vi "UMLEditor loadIniFileInfo.vi"(1 "menu":refnum<k9>, 2 "iniFile":path, 5 "error in (no error)":errorcluster) -> (11 "StabilityProblems":bool, 13 "SyncTime":u32, 15 "Ini-FileFound":bool, 16 "ToolHelp":bool, 17 "LastDiagramType":T1, 18 "FileToOpen":path, 19 "error out":errorcluster)   [LabVIEW 2014]
doc: "Gets current diagram values"
uses:
  <resource>/Framework/Providers/Open_GDS/UML/Graph_class/private/diagramType.ctl
  <resource>/Framework/Providers/Open_GDS/UML/UMLEditor/UMLEditor_SyncOptions.ctl
  <resource>/Framework/Providers/Open_GDS/UML/UMLEditor/UMLEditor_IniFileData.ctl
  <resource>/Framework/Providers/Open_GDS/UML/UMLEditor/UMLEditor_StoredPathes.ctl
  <resource>/Framework/Providers/Open_GDS/ClassProviders/Common/File/File_StoredPathesActions.ctl
  <resource>/Framework/Providers/Open_GDS/UML/UMLEditor/UMLEditor_StoredColors.ctl
  <resource>/Framework/Providers/Open_GDS/UML/UmlEditor_class/IniParamsType.ctl
  <resource>/Framework/Providers/Open_GDS/ClassProviders/Common/CommonVIs/CommonVIs_ColorMemoryAction.ctl
  <resource>/Framework/Providers/Open_GDS/UML/UMLEditor/UMLEditor MenuActionType.ctl
  <resource>/Framework/Providers/Open_GDS/UML/Graph_class/Graph.lvclass
  <resource>/Framework/Providers/Open_GDS/UML/UmlEditor_class/UmlEditor.lvclass
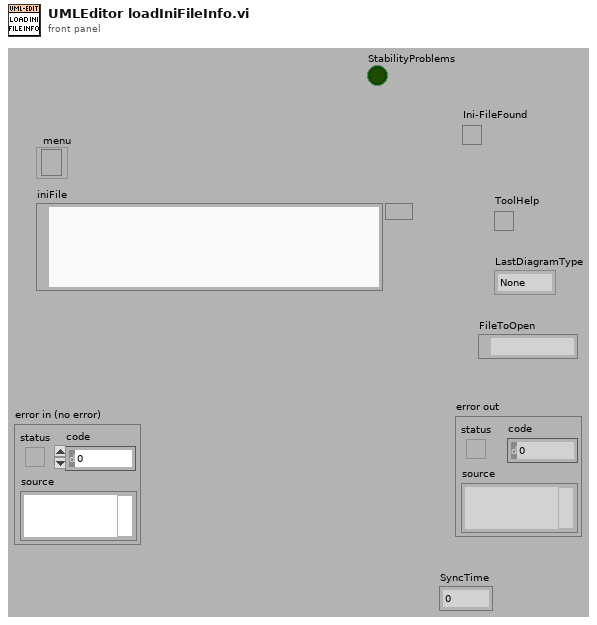
[diagram p1: front panel]
types:
  T1 = typedef "Graph.lvclass/diagramType.ctl" = enum16{"None", "Class", "Sequency", "State", "UseCase"}
  T2 = typedef "UMLEditor_IniFileData.ctl" = cluster{"RecentFiles":string[], "LastDiagramType":T1, "ShowToolHelp":bool, "Paths":cluster{"LastSerachPath":path, "QueuedArrayStateVI":path, "ClassBasePath":path, "VITemplatePath":path, "ApplicationTemplatePath":path, "RevPlugIns":path}, "Colors":cluster{"ClassBackgroudColor":u32, "ClassBackgroudColorWithClassPath":u32, "ClassBackgroudColorForApplicationVIStereotype":u32, "ClassBackgroudColorForTypeStereotype":u32, "StateBackgroudColor":u32}, "ProjectBaseClassOption":bool, "CreateTypesWhenSynchronizing":bool, "AttributeToIgnoreInSync":string[], "ToolTip":cluster{"ToolTipOpen":bool, "LastToolTip":i32}, "ClassesToIgnoreInSync":string[], "UndoSize":i32, "OpenLastSavedFile":bool, "SyncOption":T3, "SyncTime":u32, "Params":cluster{"Name":string, "Value":string}[]}
  T3 = typedef "UMLEditor_SyncOptions.ctl" = cluster{"IgnoreInstrLib":bool, "IgnoreUserLib":bool, "IgnoreViLib":bool}
  T4 = cluster{"RecentFiles":string[], "LastDiagramType":T1, "ShowToolHelp":bool, "Paths":cluster{"LastSerachPath":path, "QueuedArrayStateVI":path, "ClassBasePath":path, "VITemplatePath":path, "ApplicationTemplatePath":path, "RevPlugIns":path}, "Colors":cluster{"ClassBackgroudColor":u32, "ClassBackgroudColorWithClassPath":u32, "ClassBackgroudColorForApplicationVIStereotype":u32, "ClassBackgroudColorForTypeStereotype":u32, "StateBackgroudColor":u32}, "ProjectBaseClassOption":bool, "CreateTypesWhenSynchronizing":bool, "AttributeToIgnoreInSync":string[], "ToolTip":cluster{"ToolTipOpen":bool, "LastToolTip":i32}, "ClassesToIgnoreInSync":string[], "UndoSize":i32, "OpenLastSavedFile":bool, "SyncOption":T3}
  T5 = cluster{"RecentFiles":string[], "LastDiagramType":T1, "ShowToolHelp":bool, "Paths":cluster{"LastSerachPath":path, "QueuedArrayStateVI":path, "ClassBasePath":path, "VITemplatePath":path, "ApplicationTemplatePath":path, "RevPlugIns":path}, "Colors":cluster{"ClassBackgroudColor":u32, "ClassBackgroudColorWithClassPath":u32, "ClassBackgroudColorForApplicationVIStereotype":u32, "ClassBackgroudColorForTypeStereotype":u32, "StateBackgroudColor":u32}, "ProjectBaseClassOption":bool, "CreateTypesWhenSynchronizing":bool, "AttributeToIgnoreInSync":string[], "ToolTip":cluster{"ToolTipOpen":bool, "LastToolTip":i32}, "ClassesToIgnoreInSync":string[], "UndoSize":i32}
  T6 = cluster{"RecentFiles":string[], "LastDiagramType":T1, "ShowToolHelp":bool, "Paths":cluster{"LastSerachPath":path, "QueuedArrayStateVI":path, "ClassBasePath":path, "VITemplatePath":path, "ApplicationTemplatePath":path, "RevPlugIns":path}, "Colors":cluster{"ClassBackgroudColor":u32, "ClassBackgroudColorWithClassPath":u32, "ClassBackgroudColorForApplicationVIStereotype":u32, "ClassBackgroudColorForTypeStereotype":u32, "StateBackgroudColor":u32}, "ProjectBaseClassOption":bool, "CreateTypesWhenSynchronizing":bool, "AttributeToIgnoreInSync":string[], "ToolTip":cluster{"ToolTipOpen":bool, "LastToolTip":i32}, "ClassesToIgnoreInSync":string[], "UndoSize":i32, "OpenLastSavedFile":bool, "SyncOption":T3, "SyncTime":u32}
  T7 = typedef "UmlEditor.lvclass/IniParamsType.ctl" = enum16{"I have problem with UML stability on my computer"}
  T8 = typedef "UMLEditor_StoredColors.ctl" = enum16{"ClassBackgroudColor", "ClassBackgroudColorWithClassPath", "ClassBackgroudColorForApplicationVIStereotype", "ClassBackgroudColorForTypeStereotype", "StateBackgroudColor"}
  T9 = typedef "UMLEditor_StoredPathes.ctl" = enum16{"LastSearchPath", "QueuedArrayStateVI", "ClassBasePath", "ViTemplatePath", "ApplicationTemplatePath", "IniFilePath", "WizDir", "RevPlugInPath"}
  T10 = typedef "UMLEditor MenuActionType.ctl" = enum16{"EnableSave", "EnablePaste", "DisablePaste", "DiableSave", "AddRecentFile", "disablePropDel", "enablePropDel", "enablePropDisDel", "diasbleClassRel", "enableClassRel", "Class", "State", "Other", "EnableXMI", "DisableXMI"}
  T11 = typedef "CommonVIs_ColorMemoryAction.ctl" = enum16{"Get Color", "Set Color", "Delete Color", "Clear All Colors"}
  T12 = typedef "File_StoredPathesActions.ctl" = enum16{"Get Path", "Set Path", "Delete Path", "Clear All Paths"}
  T13 = cluster{"LastSerachPath":path, "QueuedArrayStateVI":path, "ClassBasePath":path, "VITemplatePath":path, "ApplicationTemplatePath":path, "RevPlugIns":path}
  T14 = cluster{"ClassBackgroudColor":u32, "ClassBackgroudColorWithClassPath":u32, "ClassBackgroudColorForApplicationVIStereotype":u32, "ClassBackgroudColorForTypeStereotype":u32, "StateBackgroudColor":u32}
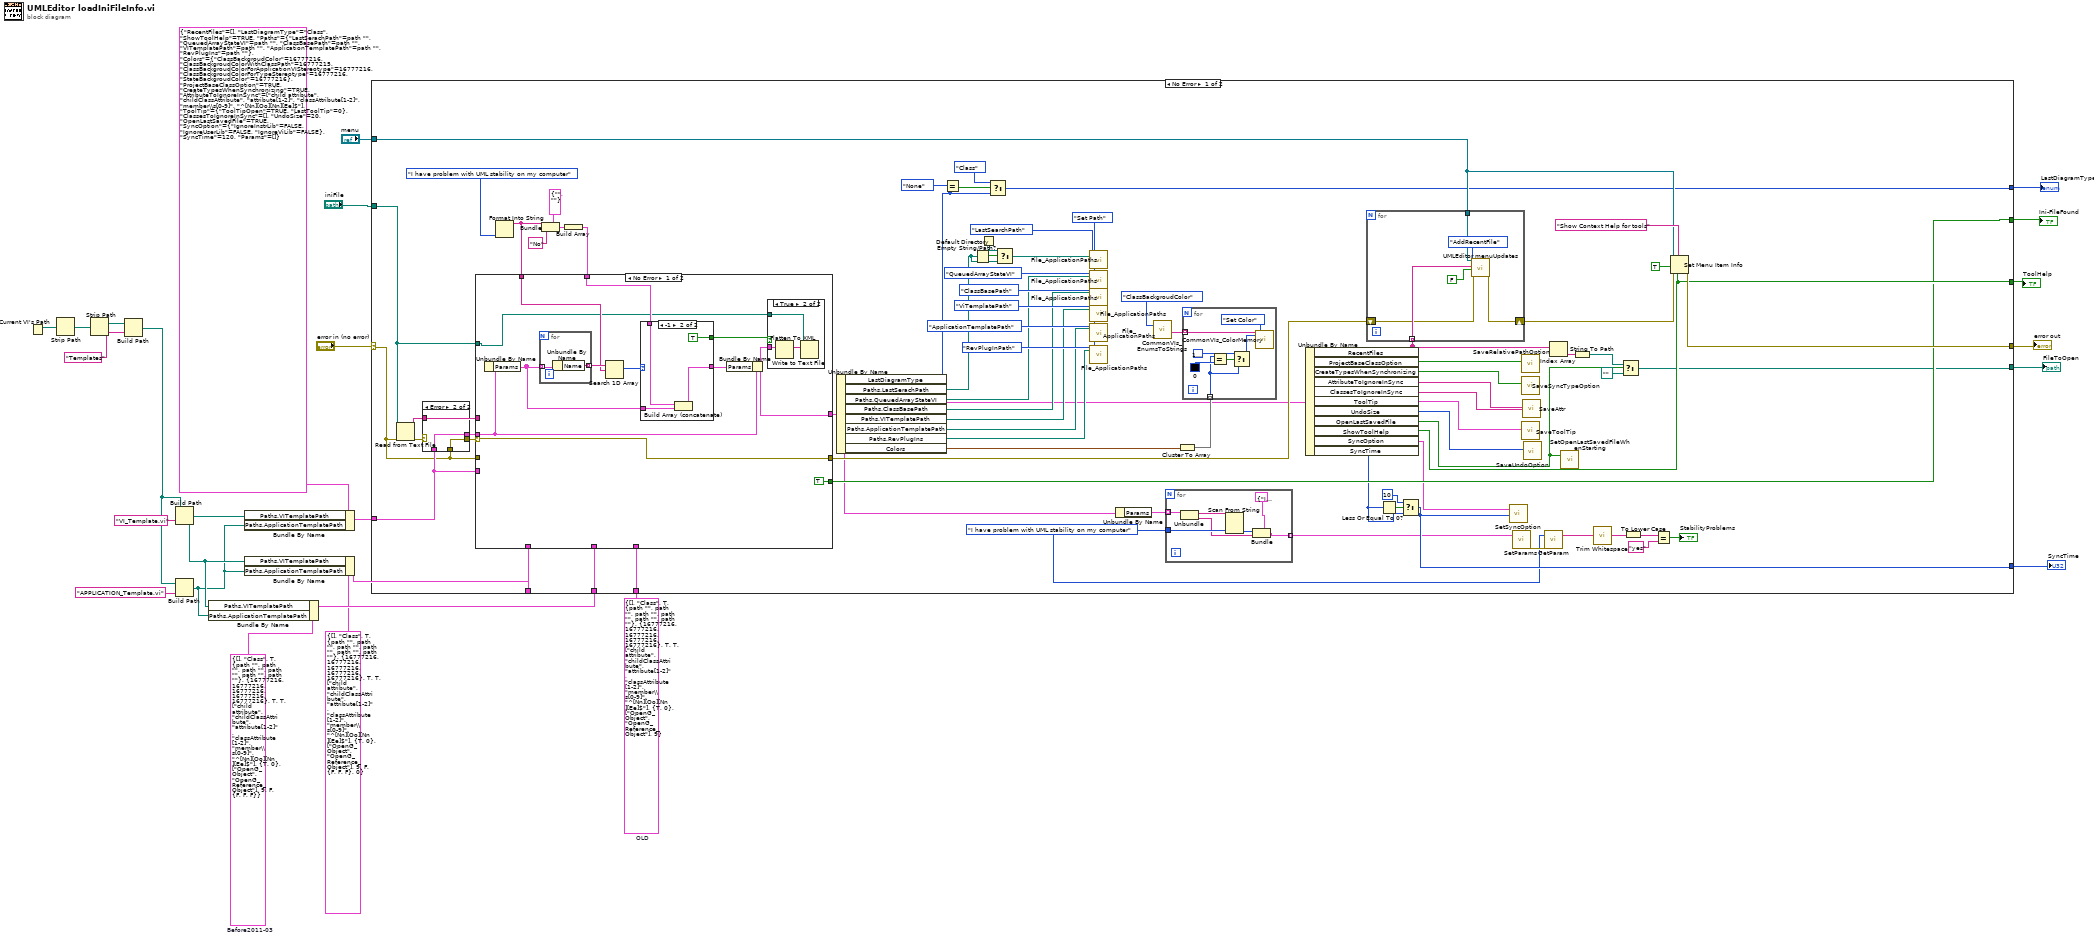
[diagram p0: block diagram]
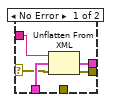
[diagram p2: hidden frame]
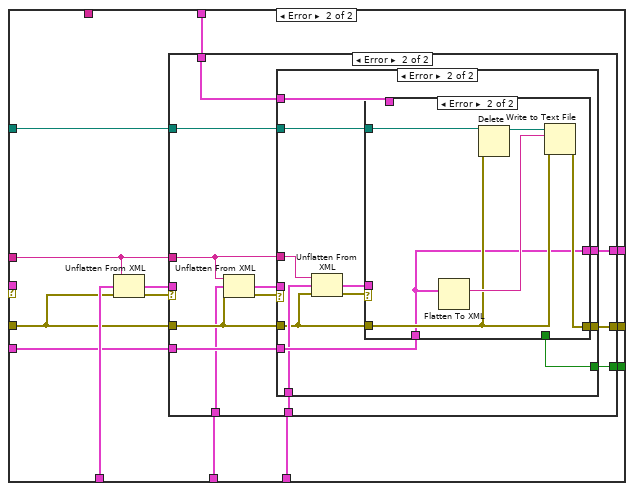
[diagram p5: hidden frame]
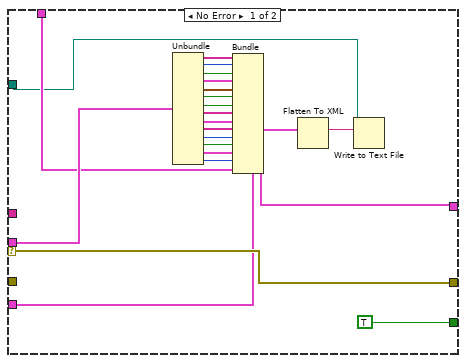
[diagram p6: hidden frame]
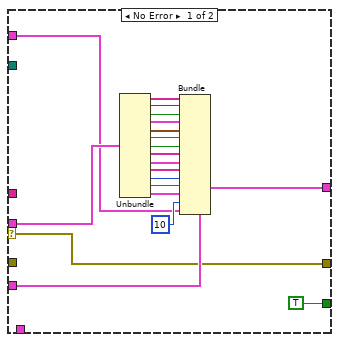
[diagram p7: hidden frame]
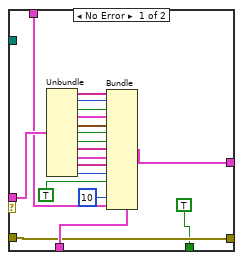
[diagram p8: hidden frame]
diagram:
  w9 = T4 {"RecentFiles"=[], "LastDiagramType"=enum."Class", "ShowToolHelp"=TRUE, "Paths"={"LastSerachPath"=path "", "QueuedArrayStateVI"=path "", "ClassBasePath"=path "", "VITemplatePath"=path "", "ApplicationTemplatePath"=path "", "RevPlugIns"=path ""}, "Colors"={"ClassBackgroudColor"=16777216, "ClassBackgroudColorWithClassPath"=16777216, "ClassBackgroudColorForApplicationVIStereotype"=16777216, "ClassBackgroudColorForTypeStereotype"=16777216, "StateBackgroudColor"=16777216}, "ProjectBaseClassOption"=TRUE, "CreateTypesWhenSynchronizing"=TRUE, "AttributeToIgnoreInSync"=["child attribute", "childClassAttribute", "attribute[1-2]", "classAttribute[1-2]", "member\\s[0-9]", "^[Nn][Oo][Nn][Ee]$"], "ToolTip"={"ToolTipOpen"=TRUE, "LastToolTip"=0}, "ClassesToIgnoreInSync"=["OpenG_Object", "OpenG_Reference_Object"], "UndoSize"=9, "OpenLastSavedFile"=FALSE, "SyncOption"={"IgnoreInstrLib"=FALSE, "IgnoreUserLib"=FALSE, "IgnoreViLib"=FALSE}}  # Before2011-03
  w11 = T5 {"RecentFiles"=[], "LastDiagramType"=enum."Class", "ShowToolHelp"=TRUE, "Paths"={"LastSerachPath"=path "", "QueuedArrayStateVI"=path "", "ClassBasePath"=path "", "VITemplatePath"=path "", "ApplicationTemplatePath"=path "", "RevPlugIns"=path ""}, "Colors"={"ClassBackgroudColor"=16777216, "ClassBackgroudColorWithClassPath"=16777216, "ClassBackgroudColorForApplicationVIStereotype"=16777216, "ClassBackgroudColorForTypeStereotype"=16777216, "StateBackgroudColor"=16777216}, "ProjectBaseClassOption"=TRUE, "CreateTypesWhenSynchronizing"=TRUE, "AttributeToIgnoreInSync"=["child attribute", "childClassAttribute", "attribute[1-2]", "classAttribute[1-2]", "member\\s[0-9]", "^[Nn][Oo][Nn][Ee]$"], "ToolTip"={"ToolTipOpen"=TRUE, "LastToolTip"=0}, "ClassesToIgnoreInSync"=["OpenG_Object", "OpenG_Reference_Object"], "UndoSize"=9}  # OLD
  n1 = Current VI's Path() -> (path=w18:path)
  n2 = Strip Path(path=w18) -> (stripped path=w17:path)  [unwired: 1 out]
  n3 = Strip Path(path=w17) -> (stripped path=w16:path)  [unwired: 1 out]
  n4 = Build Path(base path=w16, name or relative path="Templates") -> (appended path=w14:path)
  n5 = Build Path(base path=w14, name or relative path="VI_Template.vi") -> (appended path=w5:path)
  n6 = Build Path(base path=w14, name or relative path="APPLICATION_Template.vi") -> (appended path=w4:path)
  n7 = Bundle By Name(cluster=w9, "Paths.VITemplatePath"=w5, "Paths.ApplicationTemplatePath"=w4) -> (w8:T4)
  n8 = Bundle By Name(cluster=T2 {"RecentFiles"=[], "LastDiagramType"=enum."Class", "ShowToolHelp"=TRUE, "Paths"={"LastSerachPath"=path "", "QueuedArrayStateVI"=path "", "ClassBasePath"=path "", "VITemplatePath"=path "", "ApplicationTemplatePath"=path "", "RevPlugIns"=path ""}, "Colors"={"ClassBackgroudColor"=16777216, "ClassBackgroudColorWithClassPath"=16777215, "ClassBackgroudColorForApplicationVIStereotype"=16777216, "ClassBackgroudColorForTypeStereotype"=16777216, "StateBackgroudColor"=16777216}, "ProjectBaseClassOption"=TRUE, "CreateTypesWhenSynchronizing"=TRUE, "AttributeToIgnoreInSync"=["child attribute", "childClassAttribute", "attribute[1-2]", "classAttribute[1-2]", "member\\s[0-9]", "^[Nn][Oo][Nn][Ee]$"], "ToolTip"={"ToolTipOpen"=TRUE, "LastToolTip"=0}, "ClassesToIgnoreInSync"=[], "UndoSize"=20, "OpenLastSavedFile"=TRUE, "SyncOption"={"IgnoreInstrLib"=FALSE, "IgnoreUserLib"=FALSE, "IgnoreViLib"=FALSE}, "SyncTime"=120, "Params"=[]} ("INiFileData"), "Paths.VITemplatePath"=w5, "Paths.ApplicationTemplatePath"=w4) -> (w3:T2)
  n9 = Bundle By Name(cluster=T6 {"RecentFiles"=[], "LastDiagramType"=enum."Class", "ShowToolHelp"=TRUE, "Paths"={"LastSerachPath"=path "", "QueuedArrayStateVI"=path "", "ClassBasePath"=path "", "VITemplatePath"=path "", "ApplicationTemplatePath"=path "", "RevPlugIns"=path ""}, "Colors"={"ClassBackgroudColor"=16777216, "ClassBackgroudColorWithClassPath"=16777216, "ClassBackgroudColorForApplicationVIStereotype"=16777216, "ClassBackgroudColorForTypeStereotype"=16777216, "StateBackgroudColor"=16777216}, "ProjectBaseClassOption"=TRUE, "CreateTypesWhenSynchronizing"=TRUE, "AttributeToIgnoreInSync"=["child attribute", "childClassAttribute", "attribute[1-2]", "classAttribute[1-2]", "member\\s[0-9]", "^[Nn][Oo][Nn][Ee]$"], "ToolTip"={"ToolTipOpen"=TRUE, "LastToolTip"=0}, "ClassesToIgnoreInSync"=["OpenG_Object", "OpenG_Reference_Object"], "UndoSize"=9, "OpenLastSavedFile"=FALSE, "SyncOption"={"IgnoreInstrLib"=FALSE, "IgnoreUserLib"=FALSE, "IgnoreViLib"=FALSE}, "SyncTime"=0} ("INiFileData"), "Paths.VITemplatePath"=w5, "Paths.ApplicationTemplatePath"=w4) -> (w19:T6)
  n10 = case shown="No Error" "error in (no error)" {
    selector: "error in (no error)" -> [w26 w254]
    tunnel: [w101 w254] -> w24
    tunnel: [w64 _] -> w23
    tunnel: [w70 _] -> w22
    tunnel: [w80 _] -> w21
    tunnel: "menu" -> [w95 _]
    tunnel: "iniFile" -> [w81 _]
    tunnel: w19 -> [w82 _]
    tunnel: w11 -> [w60 _]
    tunnel: [w54 _] -> w10
    tunnel: w8 -> [w52 _]
    tunnel: [w49 _] -> w7
    tunnel: w3 -> [w44 _]
    frame No Error {
      w34 = IniParamsType."I have problem with UML stability on my computer" ("IniParams")
      w85 = File_StoredPathesActions."Set Path" ("Method (Get Path)")
      n11 = Read from Text File(file (use dialog)=w81, error in=w26) -> (text=w47:string, error out=w27:errorcluster)  [unwired: 4 out]
      n12 = case shown="Error" w27 {
        selector: w27 -> [w102 _]
        tunnel: w47 -> [w106 _]
        tunnel: [w105 w107] -> w46
        tunnel: [w104 w108] -> w45
        tunnel: w44 -> [w103 w108]
        tunnel: w26 -> [_ w107]
        frame No Error {
          n13 = Unflatten From XML(xml string=w106, type=w103, error in (no error)=w102) -> (value=w104:T2, error out=w105:errorcluster)
        }
        frame Error {
        }
      }
      n14 = Format Into String(IniParamsType."I have problem with UML stability on my computer" ("IniParams")) -> (resulting string=w28:string)  [unwired: 3 in, 1 out]
      n15 = Bundle(cluster=cluster{"Name":string, "Value":string} {"Name"="", "Value"=""} ("Param"), "Name"=w28, "Value"="No") -> (w40:cluster{"Name":string, "Value":string})
      n16 = Build Array(w40) -> (w39:cluster{"Name":string, "Value":string}[])
      n17 = case shown="No Error" w46 {
        selector: w46 -> [w127 _]
        tunnel: w26 -> [_ w140]
        tunnel: w82 -> [_ w149]
        tunnel: w81 -> [w117 w148]
        tunnel: [w127 w146] -> w69
        tunnel: [TRUE w145] -> w64
        tunnel: w60 -> [_ w144]
        tunnel: [w116 w143] -> w38
        tunnel: w52 -> [_ w142]
        tunnel: w47 -> [_ w141]
        tunnel: w45 -> [w123 _]
        tunnel: w44 -> [_ w139]
        tunnel: w39 -> [w120 w138]
        tunnel: w28 -> [w124 _]
        frame No Error {
          n18 = Unbundle By Name(w123) -> ("Params"=w121:cluster{"Name":string, "Value":string}[])
          n19 = for {
            tunnel: w121 -> [w137] mode=indexing
            tunnel: [w136] -> w125 mode=indexing
            n20 = Unbundle By Name(w137) -> ("Name"=w136:string)
          }
          n21 = Search 1D Array(1D array=w125, element=w124) -> (index of element=w122:i32)  [unwired: 1 in]
          n22 = case shown="-1" w122 {
            tunnel: w121 -> [w131 w135]
            tunnel: w120 -> [_ w134]
            tunnel: [w131 w133] -> w119
            tunnel: [_ TRUE] -> w118
            frame 0, Default {
            }
            frame -1 {
              n23 = Build Array (concatenate)(w134, w135) -> (w133:cluster{"Name":string, "Value":string}[])
            }
          }
          n24 = Bundle By Name(cluster=w123, "Params"=w119) -> (w116:T2)
          n25 = case shown="True" w118 {
            tunnel: w117 -> [_ w129]
            tunnel: w116 -> [_ w128]
            frame False {
            }
            frame True {
              n26 = Flatten To XML(anything=w128) -> (xml string=w130:string)
              n27 = Write to Text File(file (use dialog)=w129, text=w130) -> ()  [unwired: 1 in, 4 out]
            }
          }
        }
        frame Error {
          n28 = Unflatten From XML(xml string=w141, type=w149, error in (no error)=w140) -> (value=w147:T6, error out=w150:errorcluster)
          n29 = case shown="Error" w150 {
            selector: w150 -> [w172 _]
            tunnel: [w172 w182] -> w146
            tunnel: w140 -> [_ w178]
            tunnel: w139 -> [w155 w183]
            tunnel: w148 -> [w151 w184]
            tunnel: w147 -> [w157 _]
            tunnel: [TRUE w181] -> w145
            tunnel: w141 -> [_ w177]
            tunnel: w144 -> [_ w180]
            tunnel: [w153 w179] -> w143
            tunnel: w142 -> [_ w174]
            tunnel: w138 -> [w154 w173]
            frame No Error {
              n30 = Unbundle(w157) -> ("RecentFiles"=w170:string[], "LastDiagramType"=w169:T1, "ShowToolHelp"=w168:bool, "Paths"=w167:T13, "Colors"=w166:T14, "ProjectBaseClassOption"=w165:bool, "CreateTypesWhenSynchronizing"=w164:bool, "AttributeToIgnoreInSync"=w163:string[], "ToolTip"=w162:cluster{"ToolTipOpen":bool, "LastToolTip":i32}, "ClassesToIgnoreInSync"=w161:string[], "UndoSize"=w160:i32, "OpenLastSavedFile"=w159:bool, "SyncOption"=w158:T3, "SyncTime"=w156:u32)
              n31 = Bundle(cluster=w155, "RecentFiles"=w170, "LastDiagramType"=w169, "ShowToolHelp"=w168, "Paths"=w167, "Colors"=w166, "ProjectBaseClassOption"=w165, "CreateTypesWhenSynchronizing"=w164, "AttributeToIgnoreInSync"=w163, "ToolTip"=w162, "ClassesToIgnoreInSync"=w161, "UndoSize"=w160, "OpenLastSavedFile"=w159, "SyncOption"=w158, "SyncTime"=w156, "Params"=w154) -> (w153:T2)
              n32 = Flatten To XML(anything=w153) -> (xml string=w152:string)
              n33 = Write to Text File(file (use dialog)=w151, text=w152) -> ()  [unwired: 1 in, 4 out]
            }
            frame Error {
              n34 = Unflatten From XML(xml string=w177, type=w174, error in (no error)=w178) -> (value=w175:T4, error out=w176:errorcluster)
              n35 = case shown="Error" w176 {
                selector: w176 -> [w187 _]
                tunnel: w184 -> [_ w215]
                tunnel: w183 -> [w190 w214]
                tunnel: [w187 w213] -> w182
                tunnel: [TRUE w206] -> w181
                tunnel: w180 -> [_ w212]
                tunnel: [w188 w209] -> w179
                tunnel: w178 -> [_ w208]
                tunnel: w177 -> [_ w207]
                tunnel: w175 -> [w193 _]
                tunnel: w173 -> [w185 w205]
                frame No Error {
                  n36 = Unbundle(w193) -> ("RecentFiles"=w204:string[], "LastDiagramType"=w203:T1, "ShowToolHelp"=w202:bool, "Paths"=w201:T13, "Colors"=w200:T14, "ProjectBaseClassOption"=w199:bool, "CreateTypesWhenSynchronizing"=w198:bool, "AttributeToIgnoreInSync"=w197:string[], "ToolTip"=w196:cluster{"ToolTipOpen":bool, "LastToolTip":i32}, "ClassesToIgnoreInSync"=w195:string[], "UndoSize"=w194:i32, "OpenLastSavedFile"=w192:bool, "SyncOption"=w191:T3)
                  n37 = Bundle(cluster=w190, "RecentFiles"=w204, "LastDiagramType"=w203, "ShowToolHelp"=w202, "Paths"=w201, "Colors"=w200, "ProjectBaseClassOption"=w199, "CreateTypesWhenSynchronizing"=w198, "AttributeToIgnoreInSync"=w197, "ToolTip"=w196, "ClassesToIgnoreInSync"=w195, "UndoSize"=w194, "OpenLastSavedFile"=w192, "SyncOption"=w191, "SyncTime"=u32 10, "Params"=w185) -> (w188:T2)
                }
                frame Error {
                  n38 = Unflatten From XML(xml string=w207, type=w212, error in (no error)=w208) -> (value=w210:T5, error out=w211:errorcluster)
                  n39 = case shown="Error" w211 {
                    tunnel: w215 -> [_ w240]
                    tunnel: w214 -> [w233 w235]
                    tunnel: [w219 w236] -> w213
                    tunnel: w208 -> [w219 w237]
                    tunnel: w210 -> [w234 _]
                    tunnel: [w220 w235] -> w209
                    tunnel: [TRUE _] -> w206
                    tunnel: w205 -> [w216 _]
                    frame No Error {
                      n40 = Unbundle(w234) -> ("RecentFiles"=w232:string[], "LastDiagramType"=w231:T1, "ShowToolHelp"=w230:bool, "Paths"=w229:T13, "Colors"=w228:T14, "ProjectBaseClassOption"=w227:bool, "CreateTypesWhenSynchronizing"=w226:bool, "AttributeToIgnoreInSync"=w225:string[], "ToolTip"=w224:cluster{"ToolTipOpen":bool, "LastToolTip":i32}, "ClassesToIgnoreInSync"=w223:string[], "UndoSize"=w222:i32)
                      n41 = Bundle(cluster=w233, "RecentFiles"=w232, "LastDiagramType"=w231, "ShowToolHelp"=w230, "Paths"=w229, "Colors"=w228, "ProjectBaseClassOption"=w227, "CreateTypesWhenSynchronizing"=w226, "AttributeToIgnoreInSync"=w225, "ToolTip"=w224, "ClassesToIgnoreInSync"=w223, "UndoSize"=w222, "OpenLastSavedFile"=TRUE, "SyncTime"=u32 10, "Params"=w216) -> (w220:T2)  [unwired: 1 in]
                    }
                    frame Error {
                      n42 = Flatten To XML(anything=w235) -> (xml string=w238:string)
                      n43 = Delete(path (use dialog)=w240, error in=w237) -> (deleted path=w239:path)  [unwired: 5 out]
                      n44 = Write to Text File(file (use dialog)=w239, text=w238, error in=w237) -> (error out=w236:errorcluster)  [unwired: 3 out]
                    }
                  }
                }
              }
            }
          }
        }
      }
      n45 = Unbundle By Name(w38) -> ("LastDiagramType"=w79:T1, "Paths.LastSerachPath"=w78:path, "Paths.QueuedArrayStateVI"=w77:path, "Paths.ClassBasePath"=w76:path, "Paths.VITemplatePath"=w75:path, "Paths.ApplicationTemplatePath"=w73:path, "Paths.RevPlugIns"=w74:path, "Colors"=w72:T14)
      n46 = Equal?(x=diagramType."None" ("diagramType"), y=w79) -> (x = y?=w97:bool)
      n47 = Empty String/Path?(string/path=w78) -> (empty?=w93:bool)
      n48 = Default Directory() -> (w92:path)
      n49 = Select(t=diagramType."Class" ("diagramType"), s=w97, f=w79) -> (s? t:f=w80:T1)
      n50 = Select(t=w92, s=w93, f=w78) -> (s? t:f=w89:path)
      n51 = call <resource>:"File_ApplicationPaths.vi"("PathName"=UMLEditor_StoredPathes."LastSearchPath" ("UMLPathes"), "Path In"=w89, "Method (Get Path)"=w85) -> ()  [unwired: 1 in, 16 out]
      n52 = call <resource>:"File_ApplicationPaths.vi"("PathName"=UMLEditor_StoredPathes."QueuedArrayStateVI" ("UMLPathes"), "Path In"=w77, "Method (Get Path)"=w85) -> ()  [unwired: 1 in, 16 out]
      n53 = call <resource>:"File_ApplicationPaths.vi"("PathName"=UMLEditor_StoredPathes."ClassBasePath" ("UMLPathes"), "Path In"=w76, "Method (Get Path)"=w85) -> ()  [unwired: 1 in, 16 out]
      n54 = call <resource>:"File_ApplicationPaths.vi"("PathName"=UMLEditor_StoredPathes."ViTemplatePath" ("UMLPathes"), "Path In"=w75, "Method (Get Path)"=w85) -> ()  [unwired: 1 in, 16 out]
      n55 = call <resource>:"File_ApplicationPaths.vi"("PathName"=UMLEditor_StoredPathes."ApplicationTemplatePath" ("UMLPathes"), "Path In"=w73, "Method (Get Path)"=w85) -> ()  [unwired: 1 in, 16 out]
      n56 = call <resource>:"File_ApplicationPaths.vi"("PathName"=UMLEditor_StoredPathes."RevPlugInPath" ("UMLPathes"), "Path In"=w74, "Method (Get Path)"=w85) -> ()  [unwired: 1 in, 16 out]
      n57 = Unbundle By Name(w38) -> ("Params"=w37:cluster{"Name":string, "Value":string}[])
      n58 = call <resource>:"CommonVIs_EnumsToStrings.vi"("ArrayEnumVariantIn"=UMLEditor_StoredColors."ClassBackgroudColor" ("UMLPathes")) -> ("EnumChoices"=w83:string[])  [unwired: 2 in, 16 out]
      n59 = for {
        tunnel: w37 -> [w114] mode=indexing
        tunnel: w34 -> [w113]
        tunnel: [w109] -> w36 mode=indexing
        n60 = Unbundle(w114) -> ("Name"=w112:string, "Value"=w110:string)
        n61 = Scan From String(input string=w112, default 1=w113) -> (output 1=w111:T7)  [unwired: 3 in, 3 out]
        n62 = Bundle(cluster=cluster{"IniParams":T7, "Value":string} {"IniParams"=enum."I have problem with UML stability on my computer", "Value"=""} ("Param"), "IniParams"=w111, "Value"=w110) -> (w109:cluster{"IniParams":T7, "Value":string})
      }
      n63 = Cluster To Array(cluster=w72) -> (array=w71:u32[])
      n64 = for {
        tunnel: w83 -> [w252] mode=indexing
        tunnel: w71 -> [w247] mode=indexing
        n65 = Equal?(x=w247, y=u32 0) -> (x = y?=w250:bool)
        n66 = Select(t=u32 16777216, s=w250, f=w247) -> (s? t:f=w248:u32)
        n67 = call <resource>:"CommonVIs_ColorMemory.vi"("ColorName"=w252, "Color In"=w248, "Method (Get Color)"=CommonVIs_ColorMemoryAction."Set Color") -> ()  [unwired: 1 in, 16 out]
      }
      n68 = Unbundle By Name(w38) -> ("RecentFiles"=w58:string[], "ProjectBaseClassOption"=w68:bool, "CreateTypesWhenSynchronizing"=w67:bool, "AttributeToIgnoreInSync"=w66:string[], "ClassesToIgnoreInSync"=w62:string[], "ToolTip"=w63:cluster{"ToolTipOpen":bool, "LastToolTip":i32}, "UndoSize"=w61:i32, "OpenLastSavedFile"=w59:bool, "ShowToolHelp"=w70:bool, "SyncOption"=w53:T3, "SyncTime"=w50:u32)
      n69 = for {
        shift-right: [w246] -> w65
        shift-left: w69 -> [w241]
        tunnel: w95 -> [w245]
        tunnel: w58 -> [w244] mode=indexing
        n70 = call <resource>:"UMLEditor menuUpdates.vi"("menu"=w245, "menuAction"=UMLEditor_MenuActionType."AddRecentFile", "item"=w244, "addfirst(false)"=FALSE, "error in (no error)"=w241) -> ("error out"=w246:errorcluster)  [unwired: 1 in, 13 out]
      }
      n71 = Less Or Equal To 0?(x=w50) -> (x <= 0?=w51:bool)
      n72 = Select(t=u32 10, s=w51, f=w50) -> (s? t:f=w49:u32)
      n73 = call <resource>:"SetSyncOption.vi"("SyncOption"=w53, "SyncTime(s)"=w49) -> ()  [unwired: 17 in, 1 out]
      n74 = call <resource>:"SetParams.vi"("Params"=w36) -> ("error out"=w35:errorcluster)  [unwired: 18 in]
      n75 = call <resource>:"SaveRelativePathOption.vi"("UseProjectFolderAsBasePath"=w68) -> ()  [unwired: 1 in, 18 out]
      n76 = call <resource>:"SaveSyncTypeOption.vi"("TypeSyncOption"=w67) -> ()  [unwired: 1 in, 18 out]
      n77 = call <resource>:"SaveToolTip.vi"("ToolTip"=w63) -> ()  [unwired: 1 in, 18 out]
      n78 = call <resource>:"SaveAttr.vi"("AttrToIgnore"=w66, "ClassesToIgnore"=w62) -> ()  [unwired: 1 in, 17 out]
      n79 = call <resource>:"SaveUndoOption.vi"("UndoSize"=w61) -> ()  [unwired: 1 in, 18 out]
      n80 = call <resource>:"GetParam.vi"("IniParams"=w34, "error in (no error)"=w35) -> ("Value"=w33:string)  [unwired: 15 in, 2 out]
      n81 = Index Array(array=w58) -> (element=w57:string)  [unwired: 1 in]
      n82 = call <resource>:"SetOpenLastSavedFileWhenStarting.vi"("OpenLastSavedFileWhenStarting"=w59) -> ()  [unwired: 18 in, 1 out]
      n83 = String To Path(string=w57) -> (path=w56:path)
      n84 = call <vilib>:"Trim Whitespace.vi"("string"=w33) -> ("trimmed string"=w32:string)  [unwired: 1 in]
      n85 = Select(t=w56, s=w59, f=path "") -> (s? t:f=w54:path)
      n86 = To Lower Case(string=w32) -> (all lower case string=w31:string)
      n87 = Equal?(x=w31, y="yes") -> (x = y?=→"StabilityProblems":bool)
      n88 = Set Menu Item Info(6:w70, 7:"Show Context Help for tools" ("item tag"), 8:w65, 9:TRUE ("enabled"), 11:w95) -> (0:w101:errorcluster)  [unwired: 3 out]
    }
    frame Error {
    }
  }
  "error out" <- w24
  "Ini-FileFound" <- w23
  "ToolHelp" <- w22
  "LastDiagramType" <- w21
  "FileToOpen" <- w10
  "SyncTime" <- w7
